vi "Vacuum Pumps copy.vi"() -> ()   [LabVIEW 2011]
panel:
  out "Boolean":bool
  in  "115":bool
  in  "115 2":bool
  in  "98":bool
  in  "100":bool
  in  "102":bool
  in  "104":bool
  in  "106":bool
  in  "108 2":bool
  in  "110":bool
  in  "112":bool
  in  "97":bool
  in  "99":bool
  in  "101":bool
  in  "103":bool
  in  "105":bool
  in  "107":bool
  in  "109":bool
  in  "111":bool
  in  "114":bool
  in  "116":bool
  in  "118":bool
  in  "120":bool
  in  "122":bool
  in  "124":bool
  in  "126":bool
  in  "128":bool
  in  "113":bool
  in  "115":bool
  in  "117":bool
  in  "119":bool
  in  "121":bool
  in  "123":bool
  in  "125":bool
  in  "127":bool
  out "94":dbl
  out "93":dbl
  out "92":dbl
  out "91":dbl
  out "90":dbl
  in  "BAR94 Byte 2":u8
  in  "BAR94 Byte 1":u8
  in  "BAR93 Byte 2":u8
  in  "BAR93 Byte 1":u8
  in  "BAR92 Byte 2":u8
  in  "BAR92 Byte 1":u8
  in  "BAR91 Byte 2":u8
  in  "BAR91 Byte 1":u8
  in  "BAR90 Byte 2":u8
  in  "BAR90 Byte 1":u8
  in  "TT":bool
  in  "108":bool
  in  "107":bool
  out "Turbo Pump":bool=TRUE
  in  "105":bool
  in  "111":bool
  out "GP275 Conv.":sgl format="%#_6e"
  in  "GP354 Input Byte 2":u8
  in  "GP354 Input Byte 1":u8
  out "Ion Guage":dbl format="%#_6e"
  in  "GP275 Input Byte 1":u8
  in  "GP275 Input Byte 2":u8
  in  "GP275 Input Byte 3":u8
  in  "GP275 Input Byte 4":u8
  in  "Scroll Pump":bool=TRUE
  in  "stop":bool
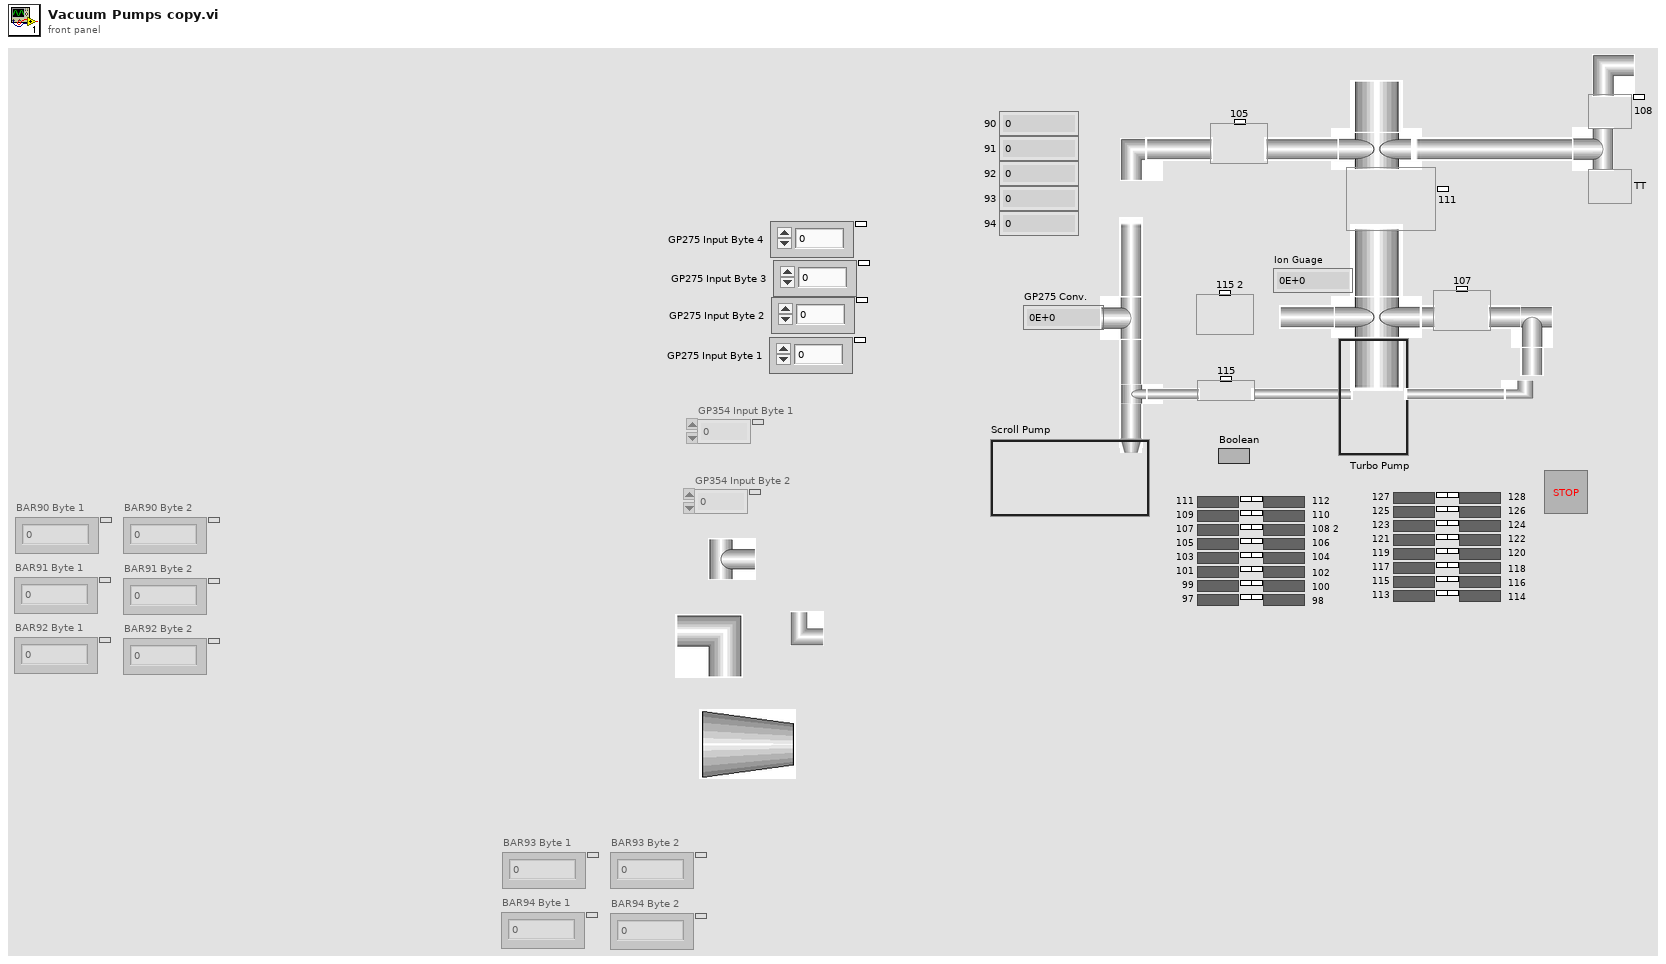
[diagram p1: front panel]
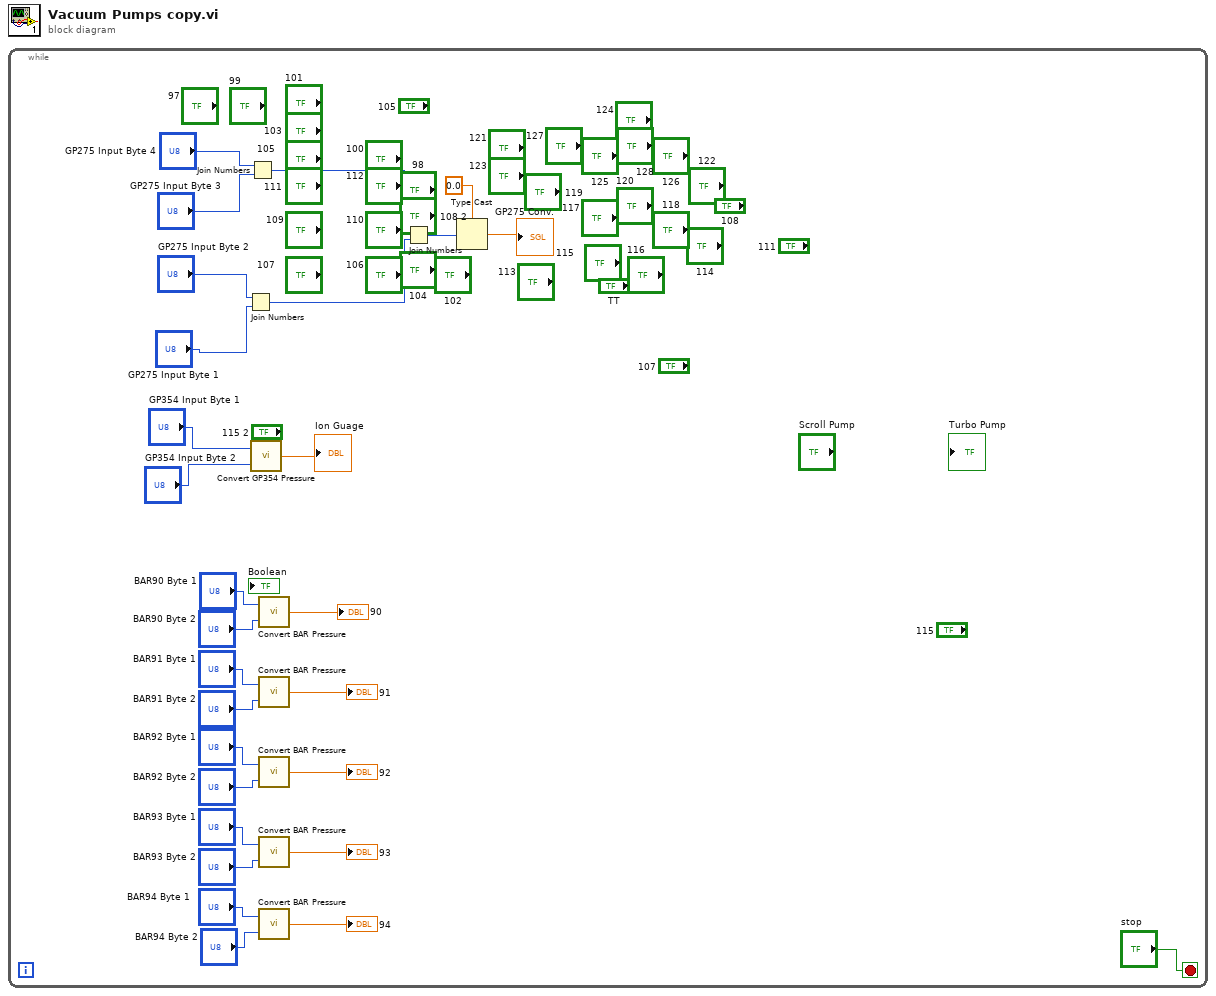
[diagram p0: block diagram]
diagram:
  n1 = while {
    stop <- "stop" stop-if-true
    n2 = Join Numbers(hi="GP275 Input Byte 2", lo="GP275 Input Byte 1") -> ((hi.lo)=w27:u16)
    n3 = Join Numbers(hi="GP275 Input Byte 4", lo="GP275 Input Byte 3") -> ((hi.lo)=w26:u16)
    n4 = call "Convert GP354 Pressure.vi"("Input Byte 2"="GP354 Input Byte 2", "Input Byte 1"="GP354 Input Byte 1") -> ("Pressure"=→"Ion Guage":dbl)
    n5 = call "Convert BAR Pressure.vi"("Input Byte 2"="BAR90 Byte 2", "Input Byte 1"="BAR90 Byte 1") -> ("Pressure"=→"90":dbl)
    n6 = call "Convert BAR Pressure.vi"("Input Byte 2"="BAR91 Byte 2", "Input Byte 1"="BAR91 Byte 1") -> ("Pressure"=→"91":dbl)
    n7 = call "Convert BAR Pressure.vi"("Input Byte 2"="BAR92 Byte 2", "Input Byte 1"="BAR92 Byte 1") -> ("Pressure"=→"92":dbl)
    n8 = call "Convert BAR Pressure.vi"("Input Byte 2"="BAR93 Byte 2", "Input Byte 1"="BAR93 Byte 1") -> ("Pressure"=→"93":dbl)
    n9 = call "Convert BAR Pressure.vi"("Input Byte 2"="BAR94 Byte 2", "Input Byte 1"="BAR94 Byte 1") -> ("Pressure"=→"94":dbl)
    n10 = Join Numbers(hi=w26, lo=w27) -> ((hi.lo)=w25:u32)
    n11 = Type Cast(type=sgl 0.0, x=w25) -> (*(type *) &x=→"GP275 Conv.":sgl)
  }
